vi "14.2 State Programming.vi"() -> ()   [LabVIEW 2019]
uses:
  13.1 DAQmx Configuration Cluster.ctl
  13.1 Weather Data.ctl
  14.1 Begining State.ctl
  <vilib>/DAQmx/read.llb/DAQmx Read (Analog DBL 1Chan 1Samp).vi
  <vilib>/DAQmx/create/channels.llb/DAQmx Create Channel (AI-Temperature-Thermocouple).vi
  <vilib>/DAQmx/miscellaneous.llb/DAQmx Fill In Error Info.vi
panel:
  in  "DAQmx Configuration Cluster":T1={"Desired Sample Rate (Hz)"=-1.0, "sample mode"=10178, "Minimum value"=-1.0, "Maximum value"=-1.0, "Thermocouple Channel"="", "units"=10143, "thermocouple type"=10072} {"thermocouple type" items=["J"=10072, "K"=10073, "N"=10077, "R"=10082, "S"=10085, "T"=10086, "B"=10047, "E"=10055]; "units" items=["Deg C"=10143, "Deg F"=10144, "Kelvins"=10325, "Deg R"=10145, "From Custom Scale"=10065]; "sample mode" items=["Finite Samples"=10178, "Continuous Samples"=10123, "Hardware Timed Single Point"=12522]}
  in  "Stop":bool
  out "Warning":string
  in  "Lower limit":dbl
  in  "Upper limit":dbl
  out "Temperature History":dbl format="%0.2f"
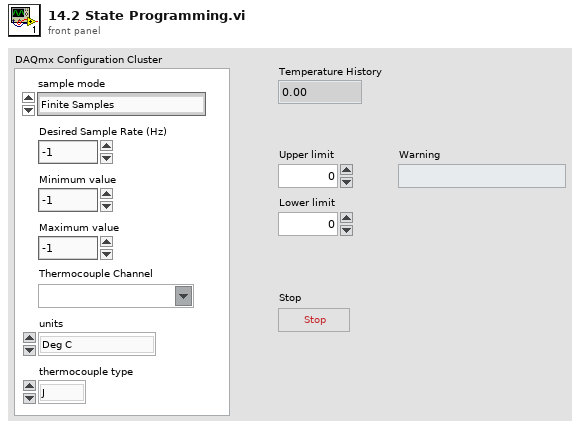
[diagram p1: front panel]
types:
  T1 = typedef "13.1 DAQmx Configuration Cluster.ctl" = cluster{"Desired Sample Rate (Hz)":dbl, "sample mode":i32, "Minimum value":dbl, "Maximum value":dbl, "Thermocouple Channel":tag, "units":i32, "thermocouple type":i32}
  T2 = typedef "14.1 Begining State.ctl" = enum16{"Initialize", "Acquire", "Analyze", "Log", "Check time", "Shutdown"}
  T3 = typedef "13.1 Weather Data.ctl" = cluster{"Current Temperature":dbl, "Max Temperature":dbl, "Min Temperature":dbl, "Warning?":bool, "Warning text":string}
  T4 = enum16{"open", "replace", "create", "open or create", "replace or create", "replace or create with confirmation"}
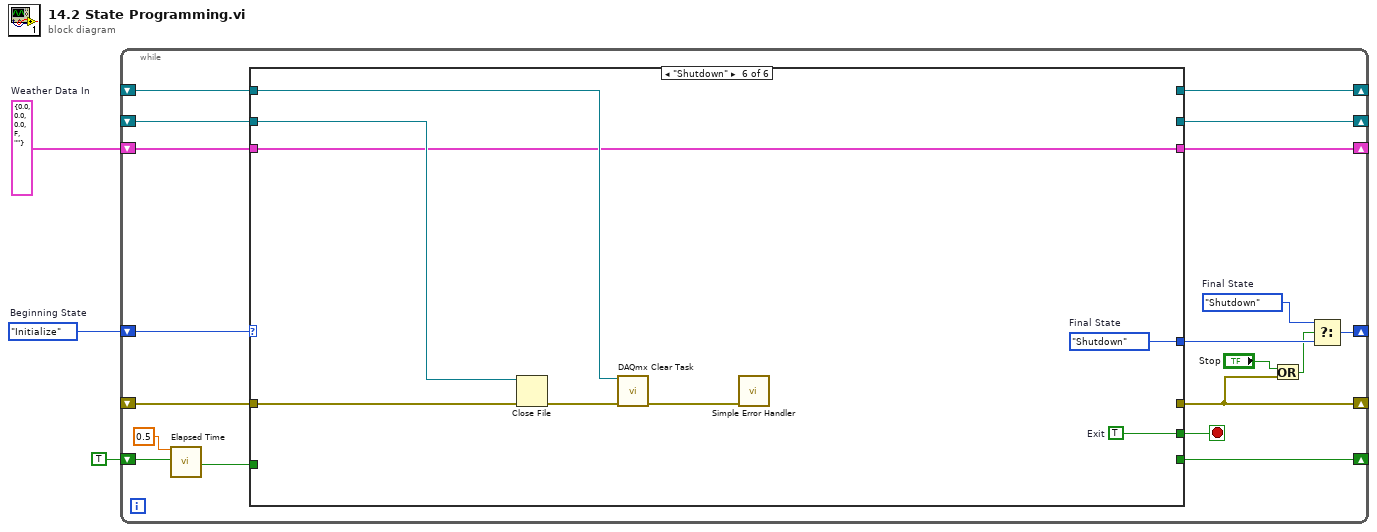
[diagram p0: block diagram]
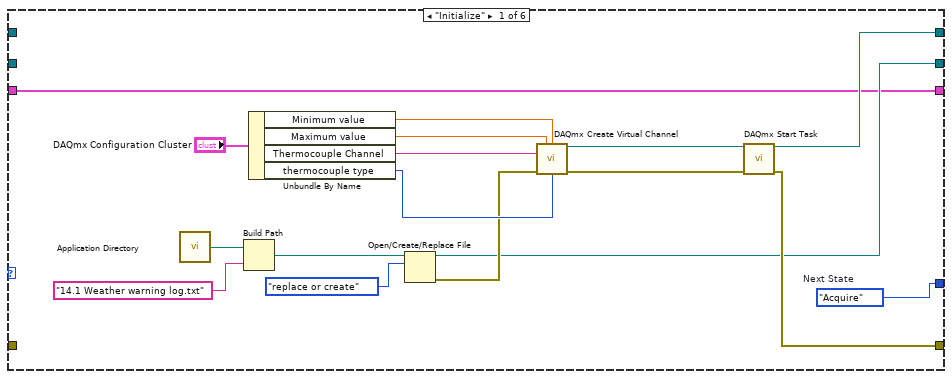
[diagram p2: hidden frame]
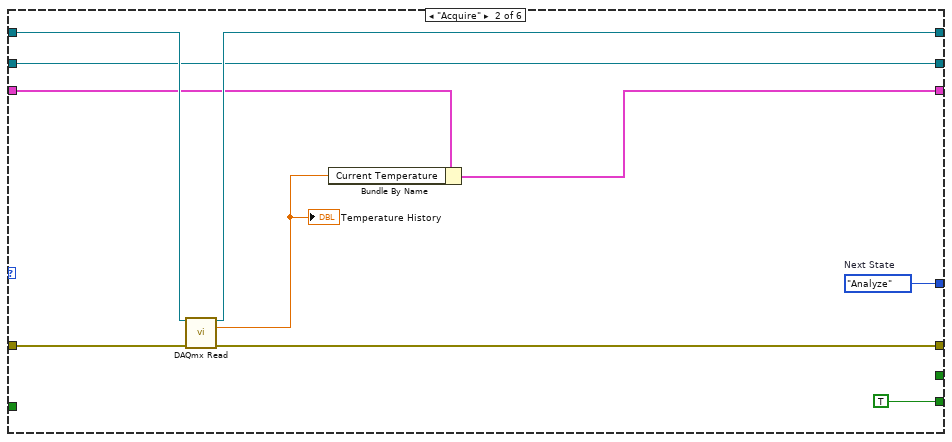
[diagram p3: hidden frame]
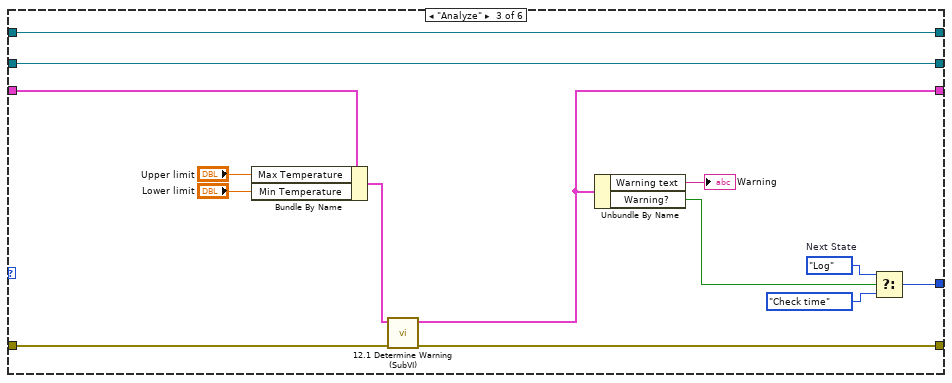
[diagram p4: hidden frame]
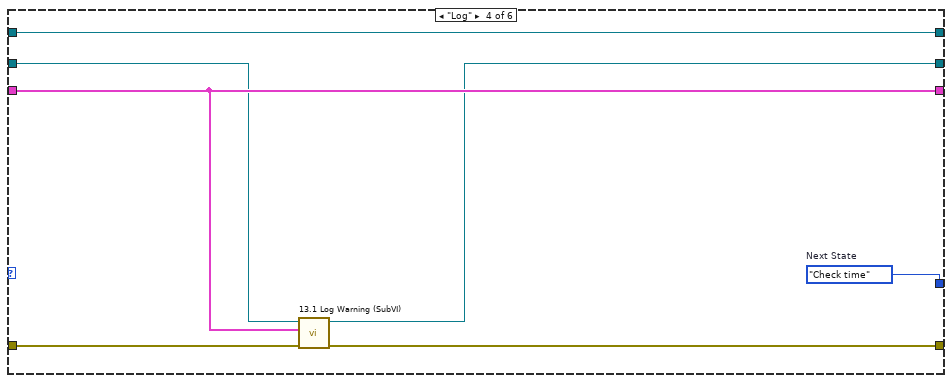
[diagram p5: hidden frame]
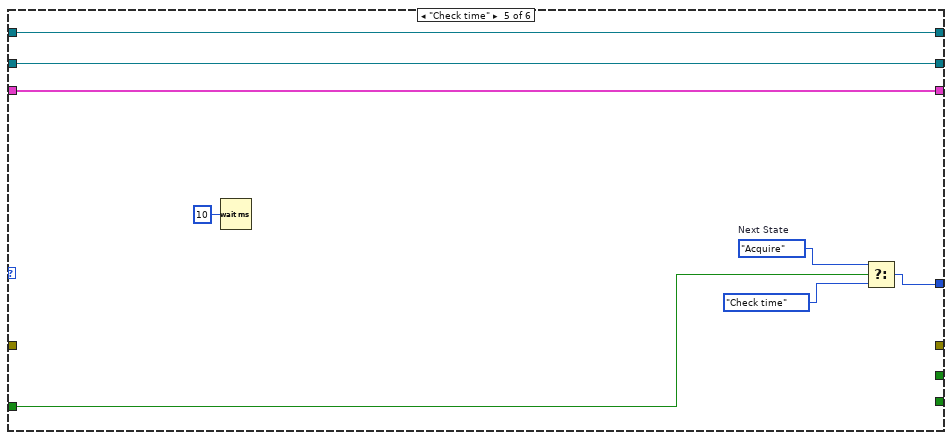
[diagram p6: hidden frame]
diagram:
  w2 = 14.1_Begining_State."Initialize"  # Beginning State
  w3 = T3 {"Current Temperature"=0.0, "Max Temperature"=0.0, "Min Temperature"=0.0, "Warning?"=FALSE, "Warning text"=""}  # Weather Data In
  n1 = while {
    shift-right: [w20] -> _
    shift-left: w3 -> [w21]
    shift-right: [w10] -> _
    shift-left: w2 -> [w22]
    shift-right: [w12] -> _
    shift-left: TRUE -> [w14]
    shift-right: [w7] -> _
    shift-left: _ -> [w19]
    shift-right: [w11] -> _
    shift-left: _ -> [w18]
    shift-right: [w16] -> _
    shift-left: _ -> [w17]
    stop <- w4 stop-if-true
    w8 = 14.1_Begining_State."Shutdown"  # Final State
    n2 = call "Elapsed Time"("Time Target (s)"=0.5, "Reset"=w14) -> ("Time has Elapsed"=w13:bool)  [unwired: 10 in, 7 out]
    n3 = case shown="\"Shutdown\"" w22 {
      tunnel: [w23 w49 w55 w65 w74 w80] -> w9
      tunnel: w21 -> [w24 w40 w63 w69 w77 w79]
      tunnel: [w24 w48 w57 w69 w77 w79] -> w20
      tunnel: w19 -> [_ w47 w60 w70 _ w83]
      tunnel: w18 -> [_ w41 w50 w68 w76 w82]
      tunnel: w17 -> [_ w46 w51 w66 w75 w81]
      tunnel: [w26 w45 w51 w66 w75 _] -> w16
      tunnel: w13 -> [_ _ _ _ w71 _]
      tunnel: [w27 w43 w58 w64 _ _] -> w7
      tunnel: [_ TRUE _ _ _ _] -> w12
      tunnel: [w25 w41 w50 w67 w76 _] -> w11
      tunnel: [_ _ _ _ _ w86] -> w4
      frame "Initialize" {
        w23 = 14.1_Begining_State."Acquire"  # Next State
        n4 = call <vilib>:"Application Directory.vi"() -> ("Application Directory"=w36:path)
        n5 = Build Path(base path=w36, name or relative path="14.1 Weather warning log.txt") -> (appended path=w38:path)
        n6 = Unbundle By Name("DAQmx Configuration Cluster") -> ("Minimum value"=w32:dbl, "Maximum value"=w30:dbl, "Thermocouple Channel"=w31:tag, "thermocouple type"=w29:i32)
        n7 = Open/Create/Replace File(file path (use dialog)=w38, operation (0:open)=T4."replace or create") -> (refnum out=w25:refnum<file>, error out=w28:errorcluster)  [unwired: 4 in, 1 out]
        n8 = call-poly <vilib>:"DAQmx Create Virtual Channel.vi"("maximum value"=w30, "minimum value"=w32, "physical channels"=w31, "error in"=w28, "thermocouple type"=w29) -> ("task out"=w34:refnum<k21>, "error out"=w33:errorcluster)  [unwired: 9 in]
        n9 = call <vilib>:"DAQmx Start Task.vi"("task/channels in"=w34, "error in"=w33) -> ("task out"=w26:refnum<k21>, "error out"=w27:errorcluster)  [unwired: 12 in]
      }
      frame "Acquire" {
        w49 = 14.1_Begining_State."Analyze"  # Next State
        n10 = call-poly <vilib>:"DAQmx Read.vi"("task/channels in"=w46, "error in"=w47) -> ("task out"=w45:refnum<k21>, "data"=w44:dbl, "error out"=w43:errorcluster)  [unwired: 11 in]
        "Temperature History" <- w44
        n11 = Bundle By Name(cluster=w40, "Current Temperature"=w44) -> (w48:T3)
      }
      frame "Analyze" {
        w54 = 14.1_Begining_State."Log"  # Next State
        n12 = Bundle By Name(cluster=w63, "Max Temperature"="Upper limit", "Min Temperature"="Lower limit") -> (w59:T3)
        n13 = call "12.1 Determine Warning (SubVI).vi"("Error In"=w60, "Weather Data In"=w59) -> ("Error Out"=w58:errorcluster, "Weather Data Out"=w57:T3)  [unwired: 8 in]
        n14 = Unbundle By Name(w57) -> ("Warning text"=→"Warning":string, "Warning?"=w52:bool)
        n15 = Select(t=w54, s=w52, f=14.1_Begining_State."Check time" ("State")) -> (s? t:f=w55:T2)
      }
      frame "Log" {
        w65 = 14.1_Begining_State."Check time"  # Next State
        n16 = call "13.1 Log Warning (SubVI).vi"("Error In"=w70, "Weather Data In"=w69, "refnum in"=w68) -> ("Error Out"=w64:errorcluster, "refnum out"=w67:refnum<file>)  [unwired: 7 in]
      }
      frame "Check time" {
        w73 = 14.1_Begining_State."Acquire"  # Next State
        n17 = Wait (ms)(milliseconds to wait=u32 10) -> ()  [unwired: 1 out]
        n18 = Select(t=w73, s=w71, f=14.1_Begining_State."Check time" ("Next State")) -> (s? t:f=w74:T2)
      }
      frame "Shutdown" {
        w80 = 14.1_Begining_State."Shutdown"  # Final State
        w86 = TRUE  # Exit
        n19 = Close File(refnum=w82, error in=w83) -> (error out=w85:errorcluster)  [unwired: 1 out]
        n20 = call <vilib>:"DAQmx Clear Task.vi"("task in"=w81, "error in"=w85) -> ("error out"=w84:errorcluster)  [unwired: 13 in]
        n21 = call <vilib>:"Simple Error Handler.vi"("error in (no error)"=w84) -> ()  [unwired: 4 in, 5 out]
      }
    }
    n22 = Or(x="Stop", y=w7) -> (x .or. y?=w6:bool)
    n23 = Select(t=w8, s=w6, f=w9) -> (s? t:f=w10:T2)
  }
